vi "Terminal_Device_Lubricate_Unit_Display.vi"   [LabVIEW 2014]
types:
  T1 = cluster{"径向油缸加载压力":u16, "轴向油缸加载压力":u16, "油箱1油液温度":u16, "润滑油温度":u16, "油箱2油液温度":u16, "试验轴承供油压力":u16, "试验轴承供油流量":u16, "陪试轴承供油流量":u16, "陪试轴承供油压力":u16, "陪试轴承供油温度":u16, "液压子系统状态字":cluster{"加载单元":cluster{"供油过滤器堵塞报警":bool, "回油过滤器堵塞报警":bool, "液位过高报警":bool, "液位过低报警":bool}, "试验轴承单元":cluster{"加热装置异常报警":bool, "油箱1液位过高报警":bool, "油箱1液位过低报警":bool, "油箱2液位过高报警":bool, "油箱2液位过低报警":bool, "供油过滤器堵塞报警":bool, "循环回路过滤器堵塞报警":bool, "回油过滤器堵塞报警":bool}, "陪试轴承单元":cluster{"供油过滤器1堵塞报警":bool, "供油过滤器2堵塞报警":bool, "回油过滤器堵塞报警":bool, "油箱液位过高报警":bool, "油箱液位过低报警":bool}}}
  T2 = cluster{"供油过滤器1堵塞报警":bool, "供油过滤器2堵塞报警":bool, "回油过滤器堵塞报警":bool, "油箱液位过高报警":bool, "油箱液位过低报警":bool}
  T3 = cluster{cluster{sgl, sgl, "陪试轴承供油流量":u16}, cluster{sgl, sgl, "陪试轴承供油压力":u16}, cluster{sgl, sgl, "陪试轴承供油温度":u16}, "陪试轴承单元":cluster{"供油过滤器1堵塞报警":bool, "供油过滤器2堵塞报警":bool, "回油过滤器堵塞报警":bool, "油箱液位过高报警":bool, "油箱液位过低报警":bool}}
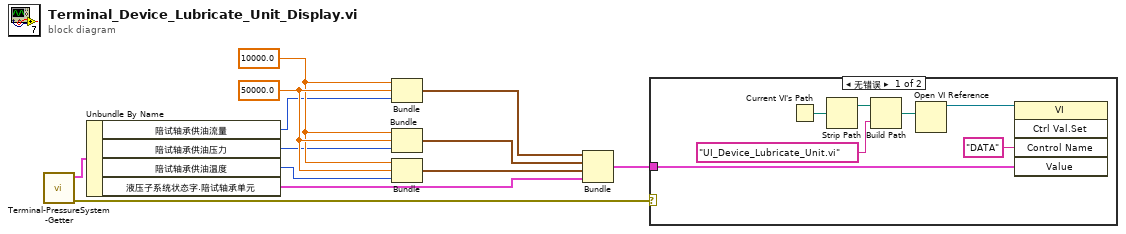
[diagram p0: block diagram]
diagram:
  w8 = sgl 50000.0
  w7 = sgl 10000.0
  n1 = call "Terminal-PressureSystem-Getter.vi"() -> ("error out"=w1:errorcluster, "设备信息"=w3:T1)  [unwired: 10 in]
  n2 = Unbundle By Name(w3) -> ("陪试轴承供油流量"=w4:u16, "陪试轴承供油压力"=w5:u16, "陪试轴承供油温度"=w6:u16, "液压子系统状态字.陪试轴承单元"=w12:T2)
  n3 = Bundle(w7, w8, "陪试轴承供油流量"=w4) -> (w9:cluster{sgl, sgl, "陪试轴承供油流量":u16})  [unwired: 1 in]
  n4 = Bundle(w7, w8, "陪试轴承供油压力"=w5) -> (w10:cluster{sgl, sgl, "陪试轴承供油压力":u16})  [unwired: 1 in]
  n5 = Bundle(w7, w8, "陪试轴承供油温度"=w6) -> (w11:cluster{sgl, sgl, "陪试轴承供油温度":u16})  [unwired: 1 in]
  n6 = Bundle(w9, w10, w11, "陪试轴承单元"=w12) -> (w2:T3)  [unwired: 1 in]
  n7 = case shown="无错误" w1 {
    tunnel: w2 -> [w13 _]
    frame No Error {
      n8 = Current VI's Path() -> (path=w17:path)
      n9 = Strip Path(path=w17) -> (stripped path=w18:path)  [unwired: 1 out]
      n10 = Build Path(base path=w18, name or relative path="UI_Device_Lubricate_Unit.vi") -> (appended path=w15:path)
      n11 = Open VI Reference(vi path=w15) -> (vi reference=w14:refnum<vi>)  [unwired: 5 in, 1 out]
      n12 = invoke class="VI" method="Ctrl Val.Set"(reference=w14, "Control Name"="DATA", "Value"=w13) -> ()  [unwired: 2 in, 5 out]
    }
    frame Error {
    }
  }
